vi "LoadCommParam.vi"(10 "section name":string) -> (2 "output cluster":T1)   [LabVIEW 2018]
uses:
  <vilib>/Utility/config.llb/Read Key (U32).vi
  <vilib>/Utility/config.llb/Read Key (String).vi
  <vilib>/Utility/config.llb/NI_LVConfig.lvlib
panel:
  out "error out":errorcluster
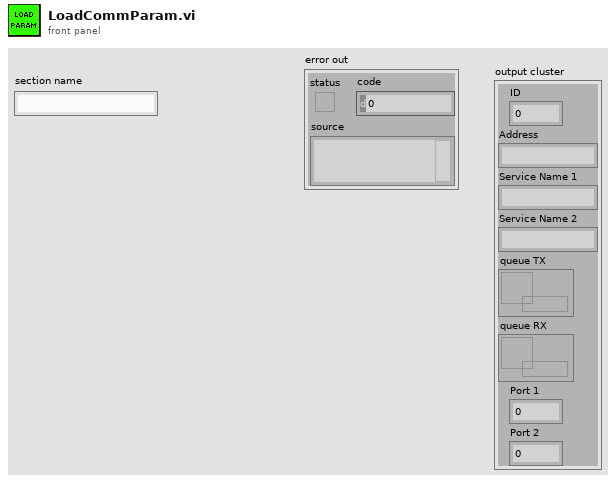
[diagram p1: front panel]
types:
  T1 = cluster{"ID":u32, "Address":string, "Service Name 1":string, "Service Name 2":string, "queue TX":refnum<queue>, "queue RX":refnum<queue>, "Port 1":u32, "Port 2":u32}
  T2 = typedef "NI_LVConfig.lvlib/Config Data RefNum.ctl" = refnum<k1>
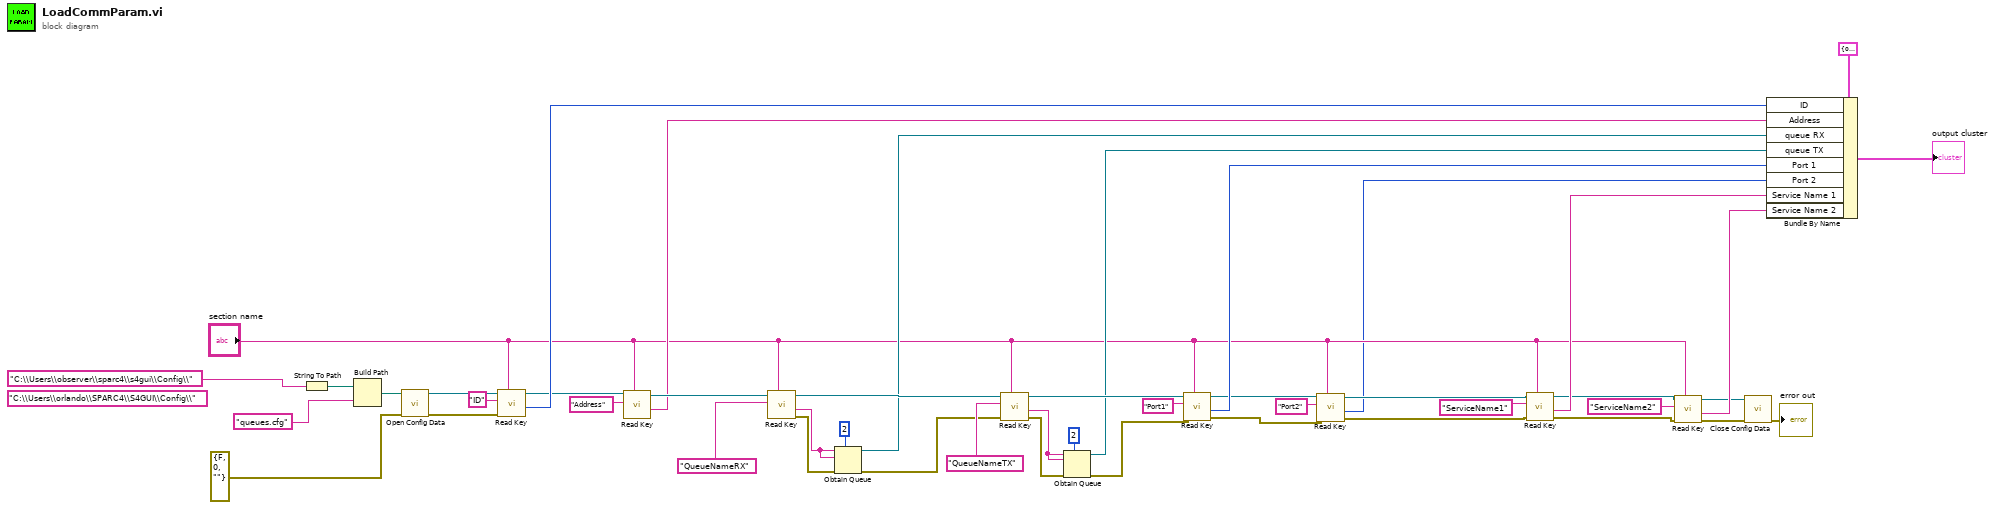
[diagram p0: block diagram]
diagram:
  (unwired) "C:\\Users\\orlando\\SPARC4\\S4GUI\\Config\\"
  n1 = String To Path(string="C:\\Users\\observer\\sparc4\\s4gui\\Config\\") -> (path=w3:path)
  n2 = Build Path(base path=w3, name or relative path="queues.cfg") -> (appended path=w47:path)
  n3 = call <vilib>:"Open Config Data.vi"("error in (no error)"=errorcluster {"status"=FALSE, "code"=0, "source"=""}, "configuration file path"=w47) -> ("error out"=w44:errorcluster, "refnum"=w46:T2)  [unwired: 7 in, 1 out]
  n4 = call-poly <vilib>:"Read Key.vi"("section"="section name", "error in (no error)"=w44, "key"="ID", "refnum"=w46) -> ("value"=w27:u32, "refnum out"=w20:T2)  [unwired: 4 in, 2 out]
  n5 = call-poly <vilib>:"Read Key.vi"("section"="section name", "key"="Address", "refnum"=w20) -> ("value"=w18:string, "refnum out"=w19:T2)  [unwired: 5 in, 2 out]
  n6 = call-poly <vilib>:"Read Key.vi"("section"="section name", "key"="QueueNameRX", "refnum"=w19) -> ("error out"=w36:errorcluster, "value"=w42:string, "refnum out"=w41:T2)  [unwired: 5 in, 1 out]
  n7 = Obtain Queue(max queue size (-1, unlimited)=2, name (unnamed)=w42, element data type=w42, error in (no error)=w36) -> (queue out=w26:refnum<queue>, error out=w35:errorcluster)  [unwired: 1 in, 1 out]
  n8 = call-poly <vilib>:"Read Key.vi"("section"="section name", "error in (no error)"=w35, "key"="QueueNameTX", "refnum"=w41) -> ("error out"=w34:errorcluster, "value"=w43:string, "refnum out"=w30:T2)  [unwired: 4 in, 1 out]
  n9 = Obtain Queue(max queue size (-1, unlimited)=2, name (unnamed)=w43, element data type=w43, error in (no error)=w34) -> (queue out=w25:refnum<queue>, error out=w31:errorcluster)  [unwired: 1 in, 1 out]
  n10 = call-poly <vilib>:"Read Key.vi"("section"="section name", "error in (no error)"=w31, "key"="Port1", "refnum"=w30) -> ("error out"=w9:errorcluster, "value"=w12:u32, "refnum out"=w7:T2)  [unwired: 4 in, 1 out]
  n11 = call-poly <vilib>:"Read Key.vi"("section"="section name", "error in (no error)"=w9, "key"="Port2", "refnum"=w7) -> ("error out"=w8:errorcluster, "value"=w4:u32, "refnum out"=w6:T2)  [unwired: 4 in, 1 out]
  n12 = call-poly <vilib>:"Read Key.vi"("section"="section name", "error in (no error)"=w8, "key"="ServiceName1", "refnum"=w6) -> ("error out"=w15:errorcluster, "value"=w24:string, "refnum out"=w17:T2)  [unwired: 4 in, 1 out]
  n13 = call-poly <vilib>:"Read Key.vi"("section"="section name", "error in (no error)"=w15, "key"="ServiceName2", "refnum"=w17) -> ("error out"=w14:errorcluster, "value"=w22:string, "refnum out"=w16:T2)  [unwired: 4 in, 1 out]
  n14 = call <vilib>:"Close Config Data.vi"("error in (no error)"=w14, "refnum"=w16) -> ("error out"=→"error out":errorcluster)  [unwired: 8 in, 1 out]
  n15 = Bundle By Name(cluster=T1 {"ID"=0, "Address"="", "Service Name 1"="", "Service Name 2"="", "queue TX"=refnum, "queue RX"=refnum, "Port 1"=0, "Port 2"=0} ("Comm Parameters"), "ID"=w27, "Address"=w18, "queue RX"=w26, "queue TX"=w25, "Port 1"=w12, "Port 2"=w4, "Service Name 1"=w24, "Service Name 2"=w22) -> (→"output cluster":T1)
